vi "CRYDisplay Unicode Boolean Text.vi"(5 "Interpret as Unicode (T)":bool, 6 "error in":errorcluster, 8 "Boolean Texts [4]":string[](array[string]), 9 "Boolean Reference":refnum<vi>) -> (0 "error out":errorcluster, 3 "Boolean Reference":refnum<vi>)   [LabVIEW 2013]
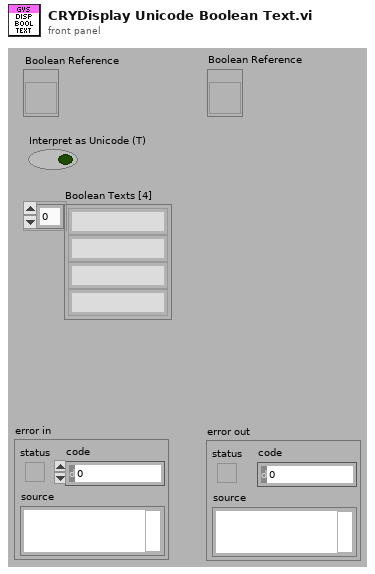
[diagram p1: front panel]
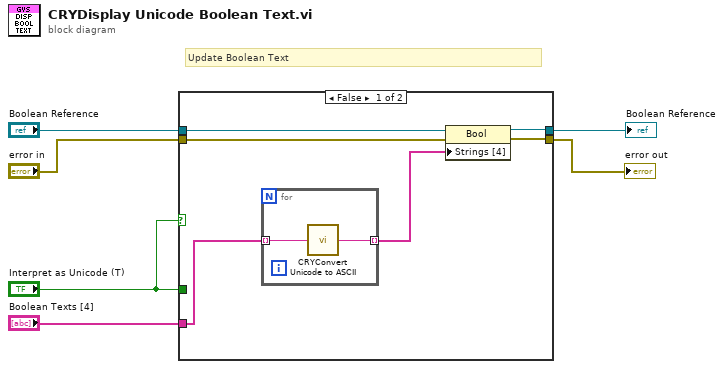
[diagram p0: block diagram]
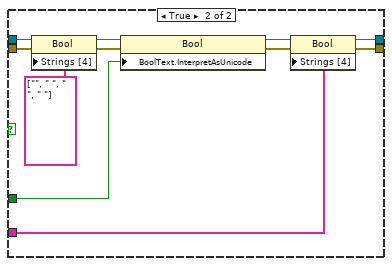
[diagram p2: hidden frame]
diagram:
  # "Update Boolean Text"
  n1 = case shown="False" "Interpret as Unicode (T)" {
    tunnel: "error in" -> [w9 w25]
    tunnel: "Boolean Reference" -> [w12 w24]
    tunnel: "Interpret as Unicode (T)" -> [_ w23]
    tunnel: "Boolean Texts [4]" -> [w8 w20]
    tunnel: [w10 w17] -> w3
    tunnel: [w11 w16] -> w2
    frame False {
      n2 = for {
        tunnel: w8 -> [w14] mode=indexing
        tunnel: [w13] -> w7 mode=indexing
        n3 = call "CRYConvert Unicode to ASCII.vi"("Unicode"=w14) -> ("ASCII"=w13:string)  [unwired: 4 in]
      }
      n4 = property class="Bool"(reference=w12, error in=w9, "Strings [4]"=w7) -> (reference out=w11:refnum<vi>, error out=w10:errorcluster)
    }
    frame True {
      n5 = property class="Bool"(reference=w24, error in=w25, "Strings [4]"=string[] ["", " ", " ", " "]) -> (reference out=w18:refnum<vi>, error out=w19:errorcluster)
      n6 = property class="Bool"(reference=w18, error in=w19, "BoolText.InterpretAsUnicode"=w23) -> (reference out=w22:refnum<vi>, error out=w21:errorcluster)
      n7 = property class="Bool"(reference=w22, error in=w21, "Strings [4]"=w20) -> (reference out=w16:refnum<vi>, error out=w17:errorcluster)
    }
  }
  "error out" <- w3
  "Boolean Reference" <- w2
